vi "DPD Apply.vi"(0 "RFmx Handle In":refnum<k21>, 1 "Selector String":string, 5 "Waveform to Predistort":T1={"Waveform Name"="Wfm", "Waveform"={"x0"=0.0, "dx"=0.0, "y"=[]}, "Signal Bandwidth (Hz)"=0.0, "PAPR (dB)"=0.0, "Burst Length (s)"=0.0, "Sample Rate"=0.0, "Burst Start Locations"=[], "Burst Stop Locations"=[], "Idle Duration Present?"=FALSE} {"Sample Rate" format="%#_6p"; "Burst Length (s)" format="%#_6p"; "PAPR (dB)" format="%.2f"; "Signal Bandwidth (Hz)" format="%.2f"; "Waveform"."y" format="%.2f"; "Waveform"."dx" format="%^.2e"; "Waveform"."x0" format="%^.2e"}, 11 "error in (no error)":errorcluster) -> (4 "RFmx Handle Out":refnum<k21>, 6 "Predistorted Waveform":T1={"Waveform Name"="Wfm", "Waveform"={"x0"=0.0, "dx"=0.0, "y"=[]}, "Signal Bandwidth (Hz)"=0.0, "PAPR (dB)"=0.0, "Burst Length (s)"=0.0, "Sample Rate"=0.0, "Burst Start Locations"=[], "Burst Stop Locations"=[], "Idle Duration Present?"=FALSE} {"Sample Rate" format="%#_6p"; "Burst Length (s)" format="%#_6p"; "PAPR (dB)" format="%.2f"; "Signal Bandwidth (Hz)" format="%.2f"; "Waveform"."y" format="%.2f"; "Waveform"."dx" format="%^.2e"; "Waveform"."x0" format="%^.2e"}, 15 "error out":errorcluster)   [LabVIEW 2016, in "RFmxSpecAn.lvlib"]
uses:
  RFmxSpecAn.lvlib
  SG/Typedefs/Waveform.ctl
  SG/SG.lvlib
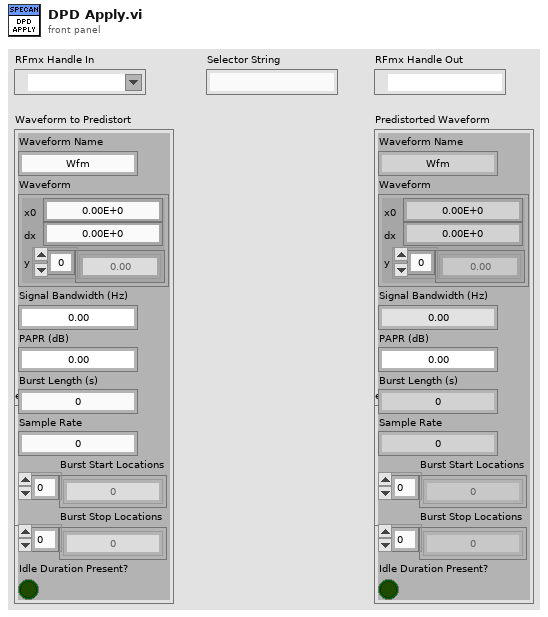
[diagram p1: front panel]
types:
  T1 = typedef "SG.lvlib/Waveform.ctl" = cluster{"Waveform Name":string, "Waveform":cluster{"x0":dbl, "dx":dbl, "y":csg[]}, "Signal Bandwidth (Hz)":dbl, "PAPR (dB)":dbl, "Burst Length (s)":dbl, "Sample Rate":dbl, "Burst Start Locations":i32[], "Burst Stop Locations":i32[], "Idle Duration Present?":bool}
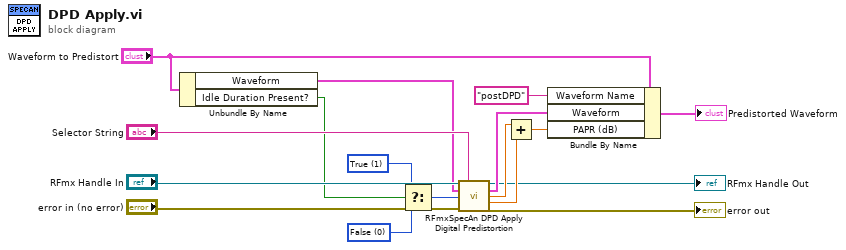
[diagram p0: block diagram]
diagram:
  w2 = 0 items=["False", "True"] ("Idle Duration Present")
  w3 = 1 items=["False", "True"] ("Idle Duration Present")
  n1 = Unbundle By Name("Waveform to Predistort") -> ("Waveform"=w9:cluster{"x0":dbl, "dx":dbl, "y":csg[]}, "Idle Duration Present?"=w1:bool)
  n2 = Select(t=w3, s=w1, f=w2) -> (s? t:f=w4:i32)
  n3 = call <vilib>:"RFmxSpecAn DPD Apply Digital Predistortion.vi"("Instrument Handle In"="RFmx Handle In", "Selector String"="Selector String", "Waveform In"=w9, "Idle Duration Present"=w4, "error in (no error)"="error in (no error)") -> ("Instrument Handle Out"=→"RFmx Handle Out":refnum<k21>, "Waveform Out"=w17:cluster{"x0":dbl, "dx":dbl, "y":csg[]}, "PAPR (dB)"=w16:dbl, "Power Offset (dB)"=w15:dbl, "error out"=→"error out":errorcluster)  [unwired: 6 in]
  n4 = Add(x=w16, y=w15) -> (x+y=w14:dbl)
  n5 = Bundle By Name(cluster="Waveform to Predistort", "Waveform Name"="postDPD", "Waveform"=w17, "PAPR (dB)"=w14) -> (→"Predistorted Waveform":T1)
